vi "Decode_Float1616.vi"(1 "Little Endian":u8[](array[numeric])) -> (0 ":16:16":dbl[](array[numeric]))   [LabVIEW 2015, in "navX Library v3.lvlib" / "navX Registry Cache.lvclass"]
uses:
  navX Registry Cache.lvclass
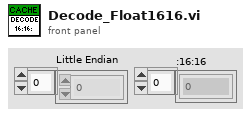
[diagram p1: front panel]
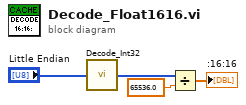
[diagram p0: block diagram]
diagram:
  n1 = call "Decode_Int32.vi"("Little Endian"="Little Endian") -> ("Int32"=w2:i32[])
  n2 = Divide(x=w2, y=65536.0) -> (x/y=→":16:16":dbl[])
